vi "R30.vi"() -> ()   [LabVIEW 2016, in "R30.lvlib"]
uses:
  R30/R30.lvlib
  Low Energy End/Low energy.lvlib
  Transmission/Transmission.lvlib
  High Energy End/High energy.lvlib
  save load/SaveLoad.lvlib
  save load/saveloadprev.ctl
panel:
  in  "Tab Control":T1(tab)
  in  "Cluster 2":T2
  out "R30 steer +X":dbl=6.705305338265999
  out "R30 steer -X":dbl=2.8585968391709997
  out "R30 steer +Y":dbl=1.425972922692
  out "R30 steer -Y":dbl=3.27987955401
  out "R30 steer +X Set":dbl=7.110598937607481
  out "R30 steer -X Set":dbl=2.889401062392519
  out "R30 steer +Y Set":dbl=3.023207629355478
  out "R30 steer -Y Set":dbl=6.976792370644522
  in  "stop":bool
  out "R30 Mag Y-steerer read":dbl=-0.4902823381440002 format="%#_3g"
  out "Mag Y-steerer range":bool=TRUE
  out "ESA range":bool=TRUE
  out "Esa Read":dbl=0.6593698178774999 min=0.0 max=200.0
  in  "ESA":dbl(slide) min=0.0 max=60.0 scale=45.0..48.0
  in  "R30 Y steerer":dbl(slide) min=-10.0 max=10.0 scale=-5.0..7.0
  in  "R30 Quad A":dbl(slide) min=0.0 max=2.0 scale=0.2..0.7
  in  "R30 X steerer":dbl(slide) min=-10.0 max=10.0 scale=-10.0..10.0
  in  "R30 Quad B":dbl(slide) min=0.0 max=2.0 scale=0.2..0.75
  out "R30 Quad A read":dbl=0.35951642376000004 min=0.0 max=200.0 format="%#_3g"
  out "R30 Quad B read":dbl=0.004890288120000014 min=0.0 max=200.0 format="%#_3g"
  out "R30 quad Range":bool=TRUE
  out "R30 Steerer X Read":dbl=3.8467084990949996 format="%#_5g"
  out "R30 Steerer Y Read":dbl=-1.853906631318 format="%#_4g"
  out "R30 Steerer range":bool=TRUE
  out "Detector cup":bool
  in  "Mag Y steerer":dbl(slide) min=-3.0 max=3.0 scale=-3.0..3.0
  in  "R30 temp file":path=path "D:/Main Tune Parameters/Temp Configs/R30.txt"
  out "SV error":errorcluster
  out "SaveLoad error":errorcluster
  # "R30"
  # "R30 Steerer Plate Voltages"
  # "Preview contains control name, conversion of variant to string, conversion of variant to double"
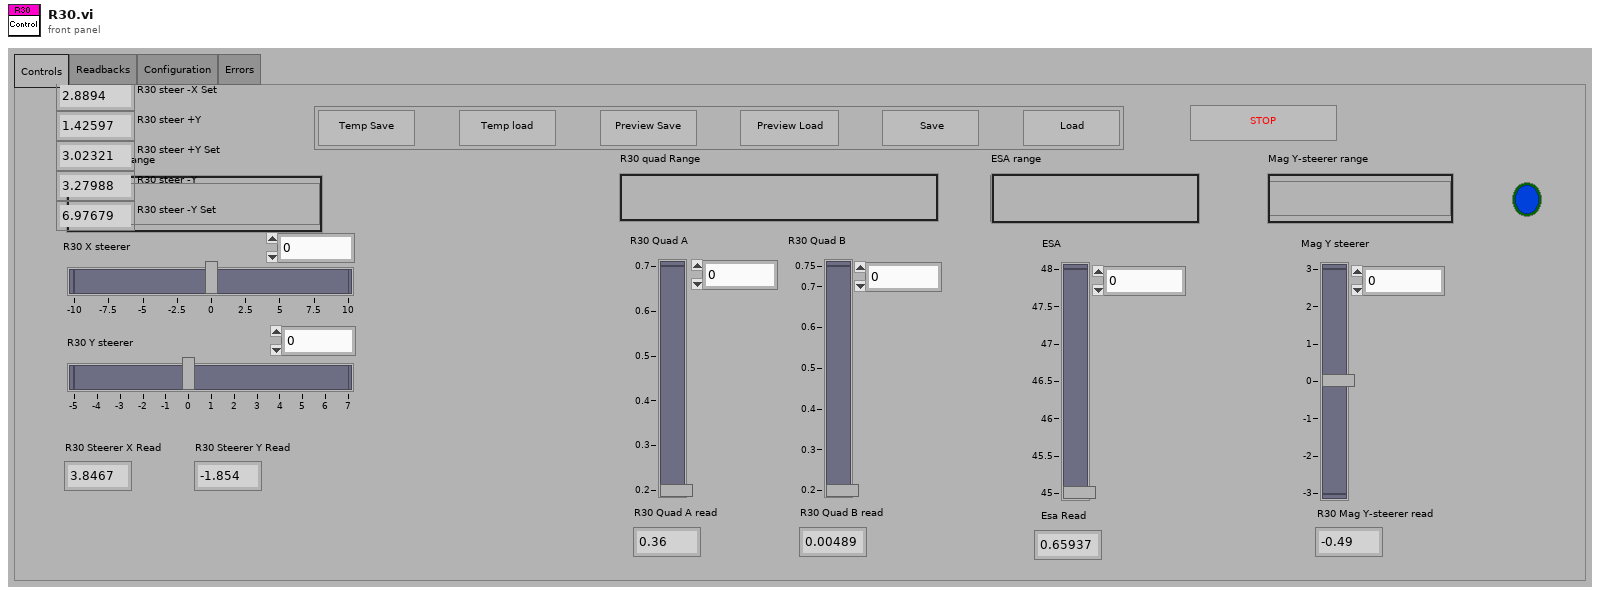
[diagram p1: front panel]
types:
  T1 = enum32{"Controls", "Readbacks", "Configuration", "Errors"}
  T2 = typedef "saveloadprev.ctl" = cluster{"Temp Save":bool, "Temp Load":bool, "Save":bool, "Load":bool, "Preview Save":bool, "Preview Load":bool}
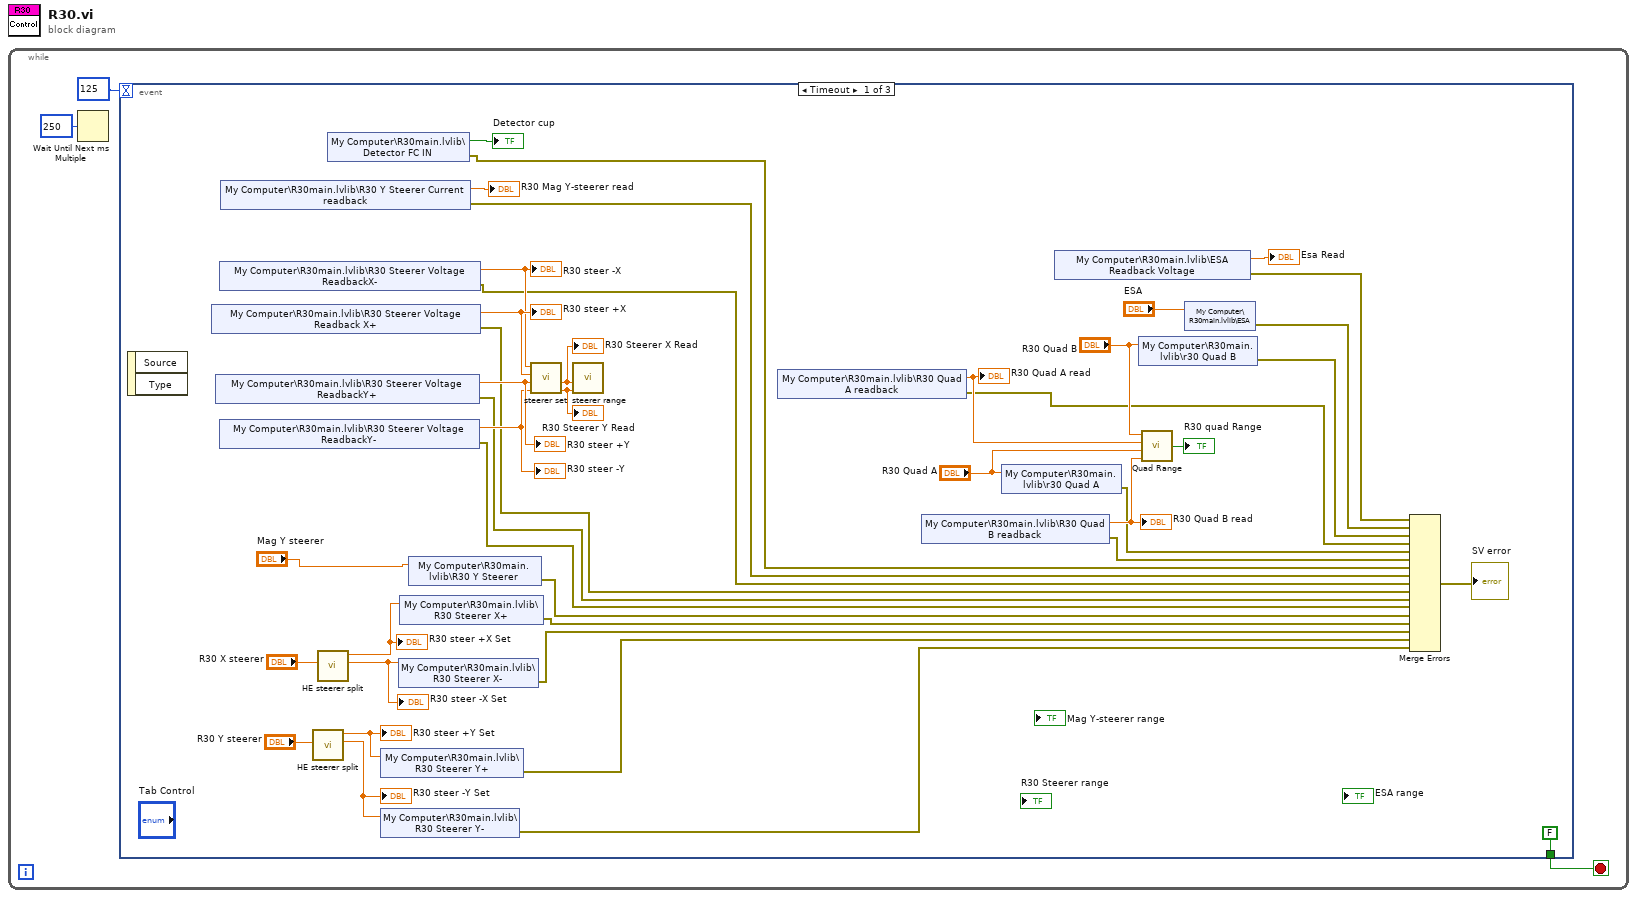
[diagram p0: block diagram]
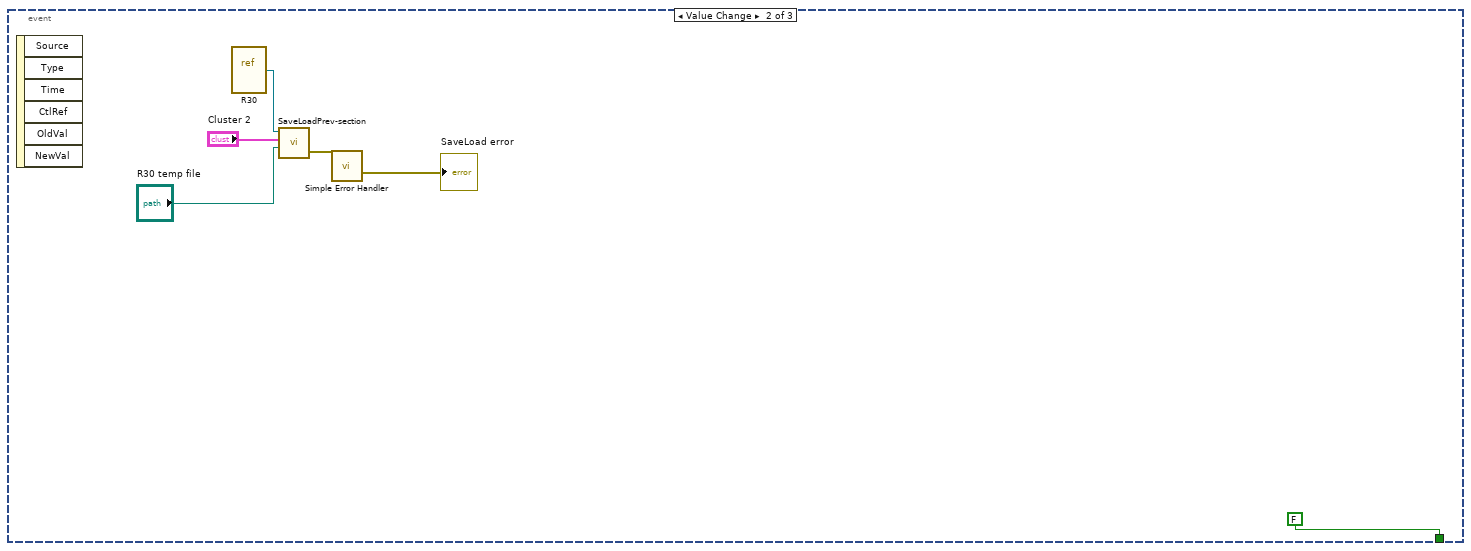
[diagram p2: hidden frame]
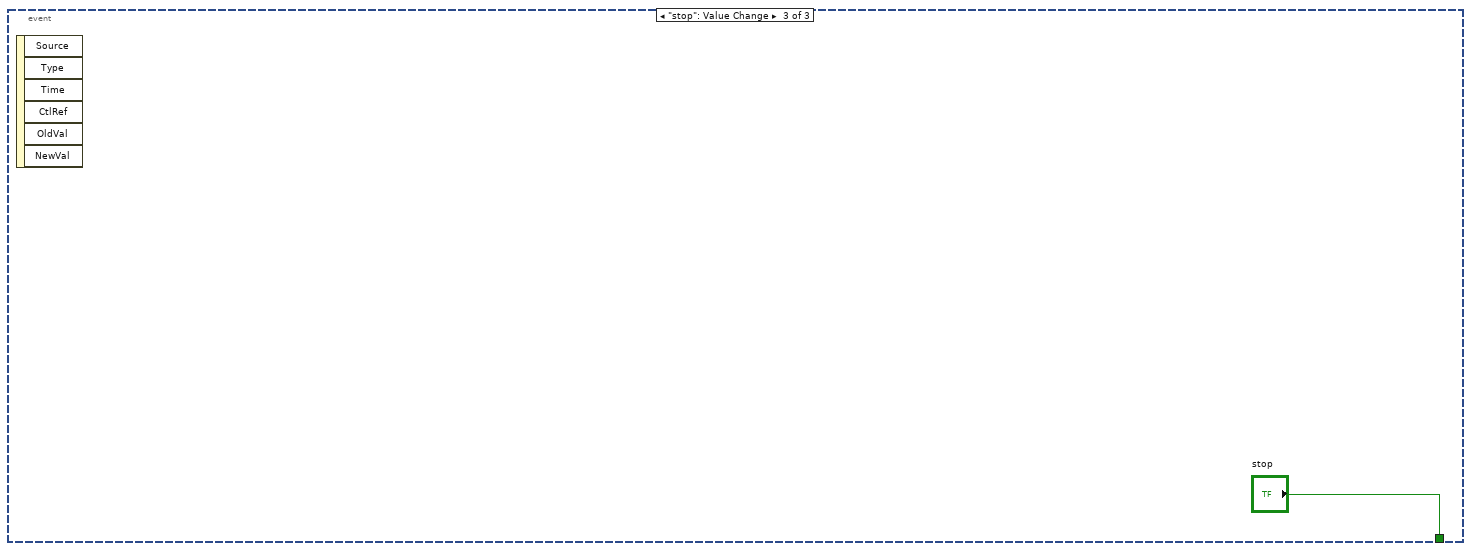
[diagram p3: hidden frame]
diagram:
  n1 = while {
    stop <- w1 stop-if-true
    n2 = Wait Until Next ms Multiple(millisecond multiple=u32 250) -> ()  [unwired: 1 out]
    n3 = event shown="[0] Timeout" {
      selector: _ -> [_ _ _]
      dyn-events: _ -> [_ _ _]
      timeout: 125 -> [_ _ _]
      tunnel: [FALSE ("stop") FALSE ("stop") "stop"] -> w1
      event Timeout {
        n4 = event-data() -> ()  [unwired: 1 in, 2 out]
        n5 = shared-variable "My Computer\\R30main.lvlib\\R30 Steerer Voltage Readback X+"() -> (w39:dbl, error out=w16:errorcluster)  [unwired: 1 in]
        "R30 steer +X" <- w39
        n6 = shared-variable "My Computer\\R30main.lvlib\\R30 Steerer Voltage ReadbackY+"() -> (w43:dbl, error out=w17:errorcluster)  [unwired: 1 in]
        "R30 steer +Y" <- w43
        n7 = shared-variable "My Computer\\R30main.lvlib\\R30 Steerer Voltage ReadbackX-"() -> (w38:dbl, error out=w15:errorcluster)  [unwired: 1 in]
        "R30 steer -X" <- w38
        n8 = shared-variable "My Computer\\R30main.lvlib\\R30 Steerer Voltage ReadbackY-"() -> (w42:dbl, error out=w18:errorcluster)  [unwired: 1 in]
        "R30 steer -Y" <- w42
        n9 = shared-variable "My Computer\\R30main.lvlib\\R30 Y Steerer Current readback"() -> (→"R30 Mag Y-steerer read":dbl, error out=w14:errorcluster)  [unwired: 1 in]
        n10 = call "HE steerer split.vi"("Steerer in"="R30 Y steerer") -> ("Steerer +"=w32:dbl, "Steerer -"=w37:dbl)  [unwired: 7 out]
        "R30 steer +Y Set" <- w32
        "R30 steer -Y Set" <- w37
        n11 = call "HE steerer split.vi"("Steerer in"="R30 X steerer") -> ("Steerer +"=w35:dbl, "Steerer -"=w36:dbl)  [unwired: 7 out]
        "R30 steer +X Set" <- w35
        "R30 steer -X Set" <- w36
        n12 = shared-variable "My Computer\\R30main.lvlib\\Detector FC IN"() -> (→"Detector cup":bool, error out=w13:errorcluster)  [unwired: 1 in]
        n13 = shared-variable "My Computer\\R30main.lvlib\\R30 Steerer Y+"(w32) -> (error out=w21:errorcluster)  [unwired: 1 in]
        n14 = shared-variable "My Computer\\R30main.lvlib\\R30 Steerer Y-"(w37) -> (error out=w22:errorcluster)  [unwired: 1 in]
        n15 = shared-variable "My Computer\\R30main.lvlib\\R30 Steerer X-"(w36) -> (error out=w20:errorcluster)  [unwired: 1 in]
        n16 = shared-variable "My Computer\\R30main.lvlib\\R30 Steerer X+"(w35) -> (error out=w19:errorcluster)  [unwired: 1 in]
        n17 = shared-variable "My Computer\\R30main.lvlib\\R30 Y Steerer"("Mag Y steerer") -> (error out=w4:errorcluster)  [unwired: 1 in]
        n18 = call "steerer set.vi"("Injector image X  -"=w38, "Injector image X +"=w39, "Injector image Y  -"=w43, "Injector image Y +"=w42) -> ("Steerer X"=w40:dbl, "Steerer Y"=w41:dbl)  [unwired: 4 out]
        "R30 Steerer X Read" <- w40
        "R30 Steerer Y Read" <- w41
        n19 = call "steerer range.vi"("Steerer Y Voltage"=w41, "Steerer X Voltage"=w40) -> ()  [unwired: 2 in, 4 out]
        n20 = shared-variable "My Computer\\R30main.lvlib\\R30 Quad A readback"() -> (w25:dbl, error out=w10:errorcluster)  [unwired: 1 in]
        "R30 Quad A read" <- w25
        n21 = shared-variable "My Computer\\R30main.lvlib\\R30 Quad B readback"() -> (w24:dbl, error out=w12:errorcluster)  [unwired: 1 in]
        "R30 Quad B read" <- w24
        n22 = shared-variable "My Computer\\R30main.lvlib\\r30 Quad A"("R30 Quad A") -> (error out=w11:errorcluster)  [unwired: 1 in]
        n23 = shared-variable "My Computer\\R30main.lvlib\\ESA Readback Voltage"() -> (→"Esa Read":dbl, error out=w7:errorcluster)  [unwired: 1 in]
        n24 = shared-variable "My Computer\\R30main.lvlib\\r30 Quad B"("R30 Quad B") -> (error out=w9:errorcluster)  [unwired: 1 in]
        n25 = call "Quad Range.vi"("Transmission Quad B read"=w24, "Transmission Quad A set"="R30 Quad A", "Transmission Quad A read"=w25, "Transmission Quad B set"="R30 Quad B") -> ("Quad range?"=→"R30 quad Range":bool)
        n26 = shared-variable "My Computer\\R30main.lvlib\\ESA"("ESA") -> (error out=w8:errorcluster)  [unwired: 1 in]
        n27 = Merge Errors(w7, w8, w9, w10, w11, w12, w13, w14, w15, w16, w17, w18, w4, w19, w20, w21, w22) -> (→"SV error":errorcluster)
      }
      event Value Change {
        n28 = event-data() -> ()  [unwired: 1 in, 6 out]
        n29 = vi-ref "R30.vi"() -> (w46:refnum<vi>)
        n30 = call "SaveLoadPrev-section.vi"("file path (use dialog)"="R30 temp file", "Cluster 2"="Cluster 2", "VI Refnum"=w46) -> ("error out"=w48:errorcluster)  [unwired: 2 in]
        n31 = call <vilib>:"Simple Error Handler.vi"("error in (no error)"=w48) -> ("error out"=→"SaveLoad error":errorcluster)  [unwired: 4 in, 4 out]
      }
      event "stop": Value Change {
        n32 = event-data() -> ()  [unwired: 1 in, 6 out]
      }
    }
  }
